vi "Acquisition Message Loop.vi"(8 "error in (no error)":errorcluster, 9 "Data Queue":refnum<queue>, 10 "Data Notifier":refnum<notifier>, 11 "Message Queues":T1) -> (0 "error out":errorcluster)   [LabVIEW 2013, in "AvaSpec Acquisition.lvlib"]
doc: "Message loop for handling messages pertaining to the acquisition of data from the hardware."
uses:
  AvaSpec Acquisition.lvlib
  support/Message Queue/All Message Queues.ctl
  support/Message Queue/Message Cluster.ctl
  Color Parameters.ctl
  Hardware Configuration.ctl
  Acquisition State.ctl
  support/Message Queue/Enqueue Message (Single).vi
  <vilib>/Utility/error.llb/Error Cluster From Error Code.vi
  <vilib>/ErrorRing/Error Ring.xnode
  support/Message Queue/AvaSpec Message Queue.lvlib
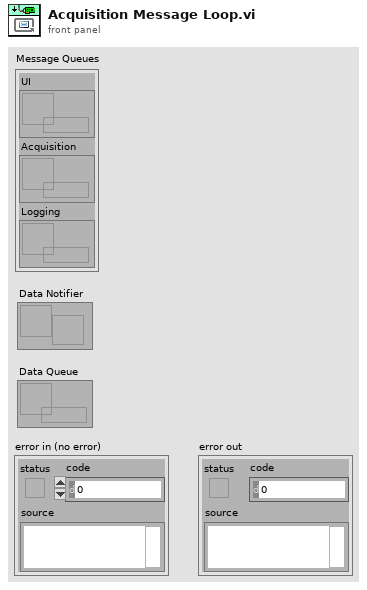
[diagram p1: front panel]
types:
  T1 = typedef "AvaSpec Message Queue.lvlib/All Message Queues.ctl" = cluster{"UI":refnum<queue>, "Acquisition":refnum<queue>, "Logging":refnum<queue>}
  T2 = typedef "AvaSpec Acquisition.lvlib/Hardware Configuration.ctl" = cluster{"Communication Settings":cluster{"Serial1":string, "Handle1":i32, "a_pDeviceId1":u8[], "a_pNumPixels":u16, "Port":i32, "a_hWnd":i32}, "a_pMeasConfig1":cluster{"StartPixel":u16, "StopPixel":u16, "IntTime":sgl, "IntDelay":u32, "NrOfAVG":u32, "DarkEnable":u8, "ForgetPercentage":u8, "SmoothPix":u16, "SmoothModel":u8, "SatDetection":u8, "TriggerMode":u8, "TriggerSource":u8, "TriggerSourceType":u8, "FlashesPerScan":u16, "LaserDelay":u32, "LaserWidth":u32, "LaserWavelenght":sgl, "RamSpectra":u16}}
  T3 = typedef "AvaSpec Acquisition.lvlib/Acquisition State.ctl" = enum16{"Idle", "Acquiring"}
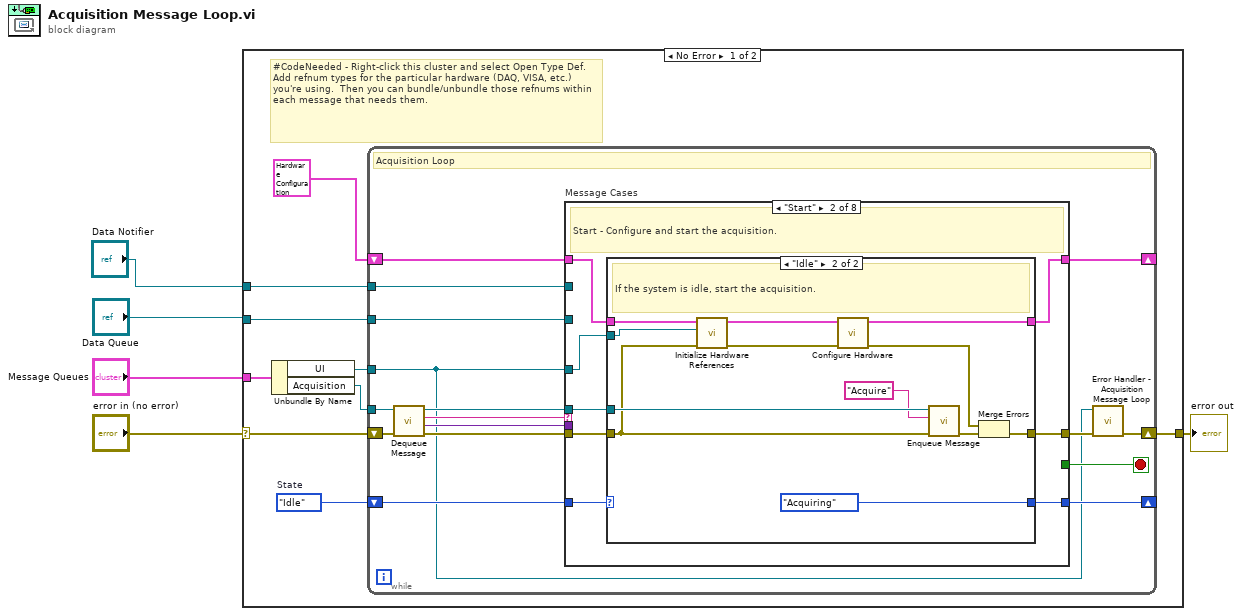
[diagram p0: block diagram]
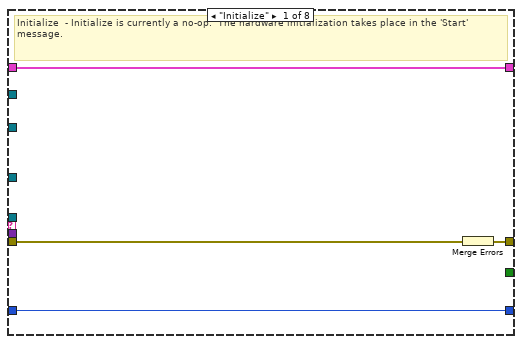
[diagram p2: hidden frame]
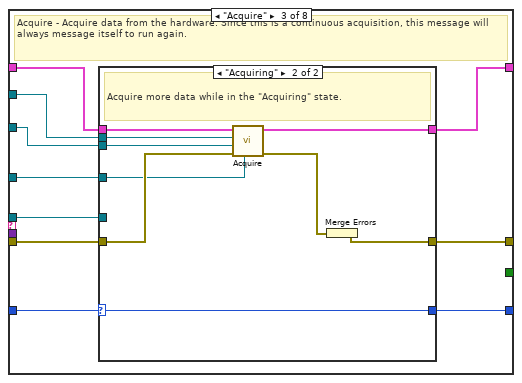
[diagram p4: hidden frame]
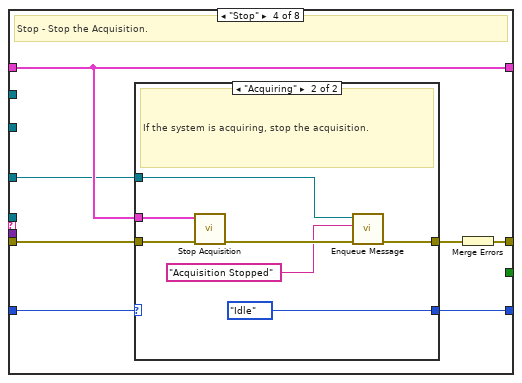
[diagram p6: hidden frame]
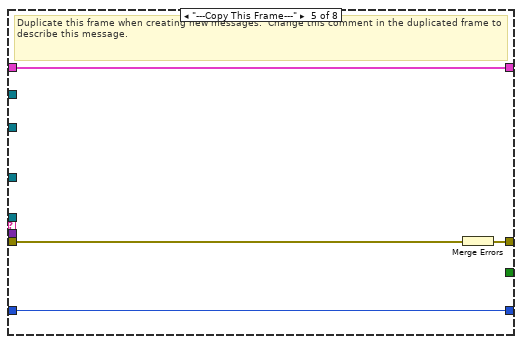
[diagram p8: hidden frame]
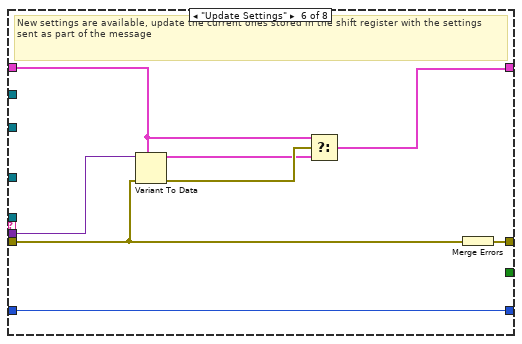
[diagram p9: hidden frame]
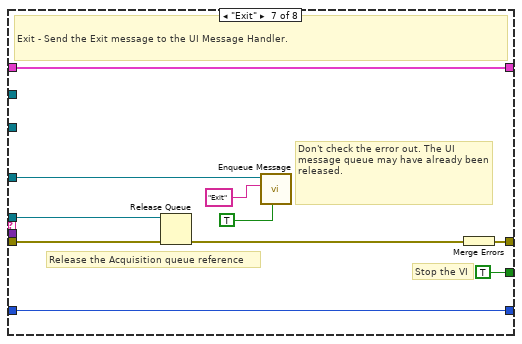
[diagram p10: hidden frame]
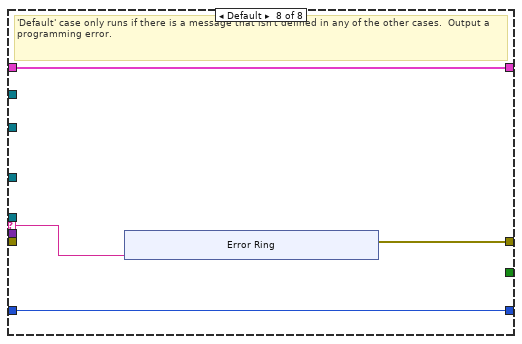
[diagram p11: hidden frame]
diagram:
  n1 = case shown="No Error" "error in (no error)" {
    selector: "error in (no error)" -> [w10 w129]
    tunnel: "Message Queues" -> [w14 _]
    tunnel: [w12 w129] -> w4
    tunnel: "Data Notifier" -> [w8 _]
    tunnel: "Data Queue" -> [w7 _]
    frame No Error {
      w6 = Acquisition_State."Idle"  # State
      # "#CodeNeeded - Right-click this cluster and select Open Type Def.  Add refnum types for the particular hardware (DAQ, VISA, etc.) you're using.  Then you can bundle/unbundle those refnums within each message that needs them."
      n2 = Unbundle By Name(w14) -> ("UI"=w9:refnum<queue>, "Acquisition"=w13:refnum<queue>)
      n3 = while {
        tunnel: w13 -> [w23]
        shift-right: [w29] -> _
        shift-left: T2 {"Communication Settings"={"Serial1"="", "Handle1"=0, "a_pDeviceId1"=[], "a_pNumPixels"=0, "Port"=0, "a_hWnd"=0}, "a_pMeasConfig1"={"StartPixel"=0, "StopPixel"=0, "IntTime"=0.0, "IntDelay"=0, "NrOfAVG"=0, "DarkEnable"=0, "ForgetPercentage"=0, "SmoothPix"=0, "SmoothModel"=0, "SatDetection"=0, "TriggerMode"=0, "TriggerSource"=0, "TriggerSourceType"=0, "FlashesPerScan"=0, "LaserDelay"=0, "LaserWidth"=0, "LaserWavelenght"=0.0, "RamSpectra"=0}} ("Data Cluster") -> [w30]
        shift-right: [w18] -> w12
        shift-left: w10 -> [w27]
        tunnel: w9 -> [w15]
        tunnel: w8 -> [w22]
        tunnel: w7 -> [w21]
        shift-right: [w19] -> _
        shift-left: w6 -> [w20]
        stop <- w28 stop-if-true
        # "Acquisition Loop"
        n4 = call "Dequeue Message.vi"("error in (no error)"=w27, "Message Queue"=w23) -> ("error out"=w26:errorcluster, "Message Data"=w24:variant, "Message"=w25:string, "dup Message Queue"=w16:refnum<queue>)  [unwired: 6 in]
        n5 = case "Message Cases" shown="\"Start\"" w25 {
          selector: w25 -> [_ _ _ _ _ _ _ w118]
          tunnel: w16 -> [_ w39 w66 _ _ _ w109 _]
          tunnel: w26 -> [w33 w40 w65 w85 w99 w101 w113 _]
          tunnel: [w34 w42 w67 w86 w97 w107 w116 w119] -> w17
          tunnel: w30 -> [w32 w41 w63 w83 w98 w103 w115 w121]
          tunnel: [w32 w38 w64 w83 w98 w102 w115 w121] -> w29
          tunnel: [_ _ _ _ _ _ TRUE _] -> w28
          tunnel: w24 -> [_ _ _ _ _ w106 _ _]
          tunnel: w15 -> [_ w35 w58 w80 _ _ w114 _]
          tunnel: w22 -> [_ _ w62 _ _ _ _ _]
          tunnel: w21 -> [_ _ w61 _ _ _ _ _]
          tunnel: w20 -> [w31 w36 w59 w82 w96 w100 w108 w120]
          tunnel: [w31 w37 w60 w81 w96 w100 w108 w120] -> w19
          frame "Initialize" {
            # "Initialize  - Initialize is currently a no-op.  The hardware initialization takes place in the 'Start' message."
            n6 = Merge Errors(w33) -> (w34:errorcluster)
          }
          frame "Start" {
            # "Start - Configure and start the acquisition."
            n7 = case shown="\"Idle\"" w36 {
              selector: w36 -> [w43 _]
              tunnel: [w44 w57] -> w42
              tunnel: w41 -> [w45 w56]
              tunnel: w40 -> [w44 w47]
              tunnel: w39 -> [_ w54]
              tunnel: [w45 w50] -> w38
              tunnel: [w43 Acquisition_State."Acquiring" ("Acquisition State")] -> w37
              tunnel: w35 -> [_ w46]
              frame "Acquiring" {
                # "The system is already acquiring. Ignore the \"Start\" message."
              }
              frame "Idle" {
                # "If the system is idle, start the acquisition."
                n8 = call "Initialize Hardware References.vi"("error in (no error)"=w47, "UI"=w46, "Hardware Resources in"=w56) -> ("error out"=w53:errorcluster, "Hardware Resources out"=w51:T2)  [unwired: 7 in]
                n9 = call "Configure Hardware.vi"("error in (no error)"=w53, "Hardware Resources in"=w51) -> ("error out"=w52:errorcluster, "Hardware Resources out"=w50:T2)  [unwired: 8 in]
                n10 = call-poly "Enqueue Message.vi"("error in (no error)"=w47, "Message"="Acquire", "Message Queue"=w54) -> ("error out"=w55:errorcluster)  [unwired: 7 in, 1 out]
                n11 = Merge Errors(w52, w55) -> (w57:errorcluster)
              }
            }
          }
          frame "Acquire" {
            # "Acquire - Acquire data from the hardware. Since this is a continuous acquisition, this message will always message itself to run again."
            n12 = case shown="\"Acquiring\"" w59 {
              selector: w59 -> [w68 w75]
              tunnel: [w69 w79] -> w67
              tunnel: w66 -> [_ _]
              tunnel: w65 -> [w69 w74]
              tunnel: [w70 w77] -> w64
              tunnel: w63 -> [w70 w76]
              tunnel: w62 -> [_ w73]
              tunnel: w61 -> [_ w72]
              tunnel: [w68 w75] -> w60
              tunnel: w58 -> [_ w71]
              frame "Idle" {
                # "Ignore \"Acquire\" messages when the acquisition is idle."
              }
              frame "Acquiring" {
                # "Acquire more data while in the \"Acquiring\" state."
                n13 = call "Acquire.vi"("UI"=w71, "error in (no error)"=w74, "Data Queue"=w72, "Data Notifier"=w73, "Hardware Resources in"=w76) -> ("error out"=w78:errorcluster, "Hardware Resources out"=w77:T2)  [unwired: 5 in]
                n14 = Merge Errors(w78) -> (w79:errorcluster)
              }
            }
          }
          frame "Stop" {
            # "Stop - Stop the Acquisition."
            n15 = case shown="\"Acquiring\"" w82 {
              selector: w82 -> [w87 _]
              tunnel: w85 -> [w88 w95]
              tunnel: [w88 w91] -> w84
              tunnel: w83 -> [_ w93]
              tunnel: [w87 Acquisition_State."Idle" ("State")] -> w81
              tunnel: w80 -> [_ w90]
              frame "Idle" {
                # "The system is already idle. Ignore the \"Stop\" message."
              }
              frame "Acquiring" {
                # "If the system is acquiring, stop the acquisition."
                n16 = call "Stop Acquisition.vi"("error in (no error)"=w95, "Hardware Resources in"=w93) -> ("error out"=w94:errorcluster)  [unwired: 9 in]
                n17 = call-poly "Enqueue Message.vi"("error in (no error)"=w94, "Message"="Acquisition Stopped", "Message Queue"=w90) -> ("error out"=w91:errorcluster)  [unwired: 7 in, 1 out]
              }
            }
            n18 = Merge Errors(w84) -> (w86:errorcluster)
          }
          frame "---Copy This Frame---" {
            # "Duplicate this frame when creating new messages.  Change this comment in the duplicated frame to describe this message."
            n19 = Merge Errors(w99) -> (w97:errorcluster)
          }
          frame "Update Settings" {
            # "New settings are available, update the current ones stored in the shift register with the settings sent as part of the message"
            n20 = Variant To Data(error in=w101, type=w103, Variant=w106) -> (data=w104:T2, error out=w105:errorcluster)
            n21 = Select(t=w103, s=w105, f=w104) -> (s? t:f=w102:T2)
            n22 = Merge Errors(w101) -> (w107:errorcluster)
          }
          frame "Exit" {
            # "Don't check the error out. The UI message queue may have already been released."
            # "Release the Acquisition queue reference"
            # "Stop the VI"
            # "Exit - Send the Exit message to the UI Message Handler."
            n23 = Release Queue(queue=w109, error in (no error)=w113) -> (error out=w110:errorcluster)  [unwired: 1 in, 2 out]
            n24 = call-poly "Enqueue Message.vi"("Priority Message? (F)"=TRUE, "Message"="Exit", "Message Queue"=w114) -> ()  [unwired: 7 in, 2 out]
            n25 = Merge Errors(w110) -> (w116:errorcluster)
          }
          frame Default {
            # "'Default' case only runs if there is a message that isn't defined in any of the other cases.  Output a programming error."
            n26 = xnode "Error Ring"("parameter 0"=w118) -> ("error out"=w119:errorcluster)
          }
        }
        n27 = call "Error Handler - Acquisition Message Loop.vi"("error in (no error)"=w17, "Message Queue"=w15) -> ("dup error in"=w18:errorcluster)  [unwired: 8 in, 1 out]
      }
    }
    frame Error {
    }
  }
  "error out" <- w4
